vi "Generate Client RPC Methods.vi"(7 "rpc method parameters":T1[](array[typedef]), 8 "error in (no error)":errorcluster, 11 "library in":refnum<vi>) -> (0 "error out":errorcluster, 3 "library out":refnum<vi>)   [LabVIEW 2019, in "gRPC Template Creation Utility.lvlib"]
uses:
  gRPC Template Creation Utility.lvlib
  TypeDefs/RPC Method Parameters.ctl
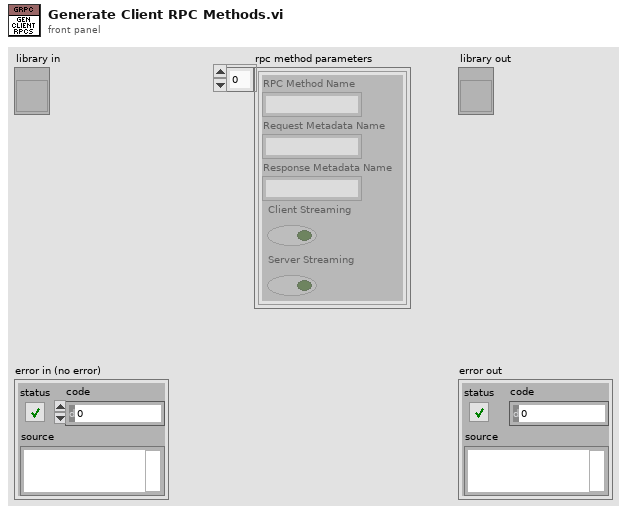
[diagram p1: front panel]
types:
  T1 = typedef "gRPC Template Creation Utility.lvlib/RPC Method Parameters.ctl" = cluster{"RPC Method Name":string, "Request Metadata Name":string, "Response Metadata Name":string, "Client Streaming":bool, "Server Streaming":bool}
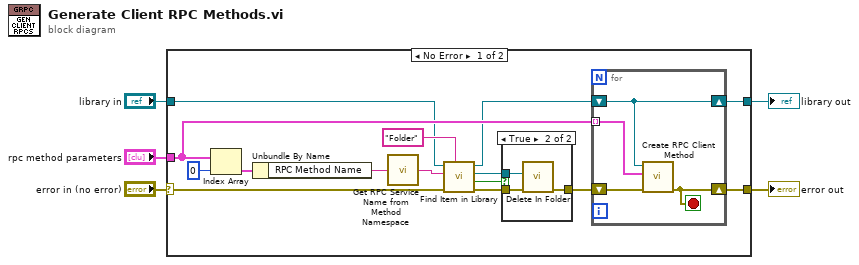
[diagram p0: block diagram]
diagram:
  n1 = case shown="No Error" "error in (no error)" {
    selector: "error in (no error)" -> [w12 w30]
    tunnel: [w20 w30] -> w5
    tunnel: "library in" -> [w8 w29]
    tunnel: [w19 w29] -> w2
    tunnel: "rpc method parameters" -> [w18 _]
    frame No Error {
      n2 = Index Array(array=w18, index=0) -> (element=w16:T1)
      n3 = Unbundle By Name(w16) -> ("RPC Method Name"=w15:string)
      n4 = call "Get RPC Service Name from Method Namespace.vi"("RPC Method Name"=w15) -> ("RPC Service Name"=w14:string)
      n5 = call "Find Item in Library.vi"("Item Type"="Folder", "error in (no error)"=w12, "Item Name"=w14, "Library item in"=w8) -> ("error out"=w11:errorcluster, "Found?"=w9:bool, "Project Item (Library Item)"=w6:refnum<vi>, "Library item out"=w7:refnum<vi>)  [unwired: 4 in]
      n6 = case shown="True" w9 {
        tunnel: [w21 w23] -> w10
        tunnel: w11 -> [w21 w24]
        tunnel: w6 -> [_ w22]
        frame False {
        }
        frame True {
          n7 = call "Delete In Folder.vi"("error in (no error)"=w24, "ProjectItem in"=w22) -> ("error out"=w23:errorcluster)  [unwired: 9 in]
        }
      }
      n8 = for {
        tunnel: w18 -> [w25] mode=indexing
        shift-right: [w26] -> w20
        shift-left: w10 -> [w28]
        shift-right: [w27] -> w19
        shift-left: w7 -> [w27]
        stop <- w26 stop-if-true
        n9 = call "Create RPC Client Method.vi"("error in (no error)"=w28, "rpc method parameters"=w25, "library in"=w27) -> ("error out"=w26:errorcluster)  [unwired: 7 in, 1 out]
      }
    }
    frame Error {
    }
  }
  "error out" <- w5
  "library out" <- w2
